vi "NewtonsPSM_Conf_VVM.vi"(4 "LVDT Scale Factor (0,1)":dbl=0.1 min=0.0 max=10000.0 step=0.01, 5 "Upper Limit (1)":dbl=1.0 min=1.0 step=0.1, 6 "Offset (0°)":dbl min=-360.0 max=360.0 step=0.01, 7 "Parameter (In Phase)":u16(ring) items=["In Phase", "Quadrature", "Tan d", "Magnitude", "Phase", "In-Phase Ratio", "RMS", "RMS2/RMS1", "LVDT Diff", "LVDT Ratio"], 8 "error in (no error)":errorcluster, 10 "Null meter (Off)":u16(ring) items=["OFF", "Auto", "Manual"], 11 "VISA session":refnum<visa-resource-name>) -> (0 "error out":errorcluster, 3 "dup VISA session":refnum<visa-resource-name>)   [LabVIEW 2025, in "NewtonsPSM1735.lvlib"]
doc: "This VI set the Integration parameters for the PPA2530."
uses:
  NewtonsPSM1735.lvlib
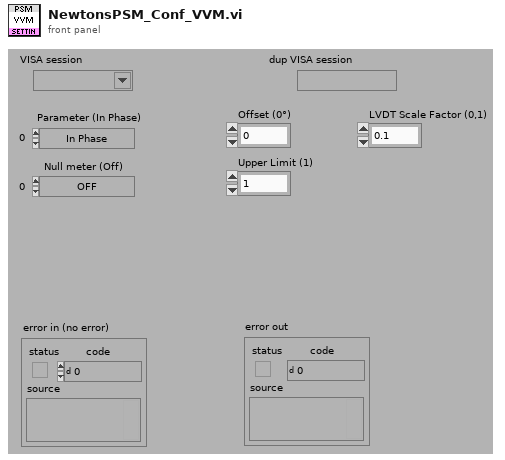
[diagram p1: front panel]
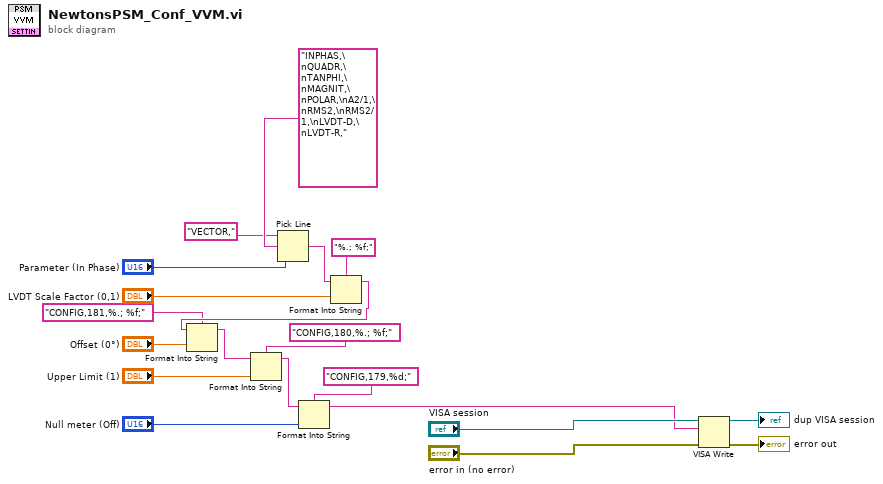
[diagram p0: block diagram]
diagram:
  n1 = Pick Line(string ("")="VECTOR,", multi-line string="INPHAS,\nQUADR,\nTANPHI,\nMAGNIT,\nPOLAR,\nA2/1,\nRMS2,\nRMS2/1,\nLVDT-D,\nLVDT-R,", line index="Parameter (In Phase)") -> (output string=w13:string)
  n2 = Format Into String(format string="%.; %f;" ("chaîne de format"), initial string=w13, "LVDT Scale Factor (0,1)") -> (resulting string=w9:string)  [unwired: 1 in, 1 out]
  n3 = Format Into String(format string="CONFIG,181,%.; %f;" ("chaîne de format"), initial string=w9, "Offset (0°)") -> (resulting string=w6:string)  [unwired: 1 in, 1 out]
  n4 = Format Into String(format string="CONFIG,180,%.; %f;" ("chaîne de format"), initial string=w6, "Upper Limit (1)") -> (resulting string=w3:string)  [unwired: 1 in, 1 out]
  n5 = Format Into String(format string="CONFIG,179,%d;" ("chaîne de format"), initial string=w3, "Null meter (Off)") -> (resulting string=w1:string)  [unwired: 1 in, 1 out]
  n6 = VISA Write(VISA resource name="VISA session", write buffer=w1, error in (no error)="error in (no error)") -> (VISA resource name out=→"dup VISA session":refnum<visa-resource-name>, error out=→"error out":errorcluster)  [unwired: 1 out]
